vi "MultiplotGraph.vi"() -> ()   [LabVIEW 2018]
panel:
  in  "Squrewave \nfrequency":dbl(slide) scale=0.0..10.0
  in  "Sinewave \nfrequency":dbl(slide) scale=0.0..10.0
  in  "stop":bool
  out "Waveform Graph":dynamicdata(graph)
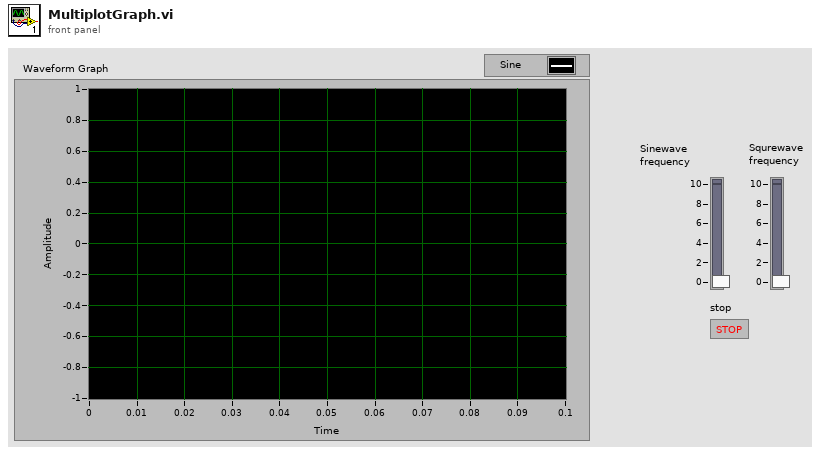
[diagram p1: front panel]
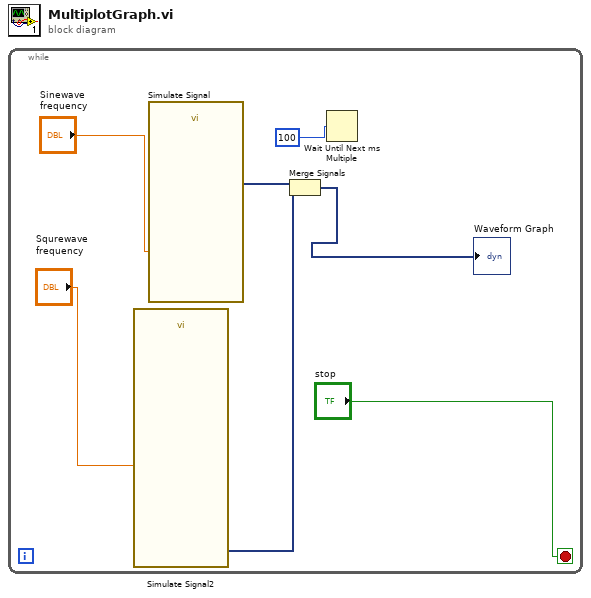
[diagram p0: block diagram]
diagram:
  n1 = while {
    stop <- "stop" stop-if-true
    n2 = call "Simulate Signal2"("Frequency"="Squrewave \nfrequency") -> ("Square"=w2:dynamicdata)  [unwired: 13 in, 1 out]
    n3 = call "Simulate Signal"("Frequency"="Sinewave \nfrequency") -> ("Sine"=w4:dynamicdata)  [unwired: 13 in, 1 out]
    n4 = Merge Signals(w4, w2) -> (→"Waveform Graph":dynamicdata)
    n5 = Wait Until Next ms Multiple(millisecond multiple=100) -> ()  [unwired: 1 out]
  }
